vi "set_translation_style.vi"(8 "error in (no error)":errorcluster, 10 "translation style":enum16{"relative", "absolute"}(ring), 11 "StageDL090409Scaffold in":refnum<class "StageDL090409Scaffold.lvclass">) -> (0 "error out":errorcluster, 3 "StageDL090409Scaffold out":refnum<class "StageDL090409Scaffold.lvclass">)   [LabVIEW 2010, in "StageDL090409Scaffold.lvclass"]
uses:
  StageDL090409Scaffold.lvclass
  StageDL090409Scaffold.lvclass/StageDL090409Scaffold.ctl
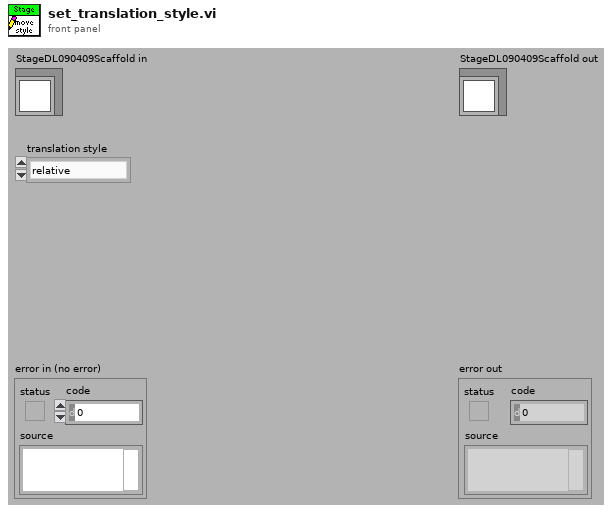
[diagram p1: front panel]
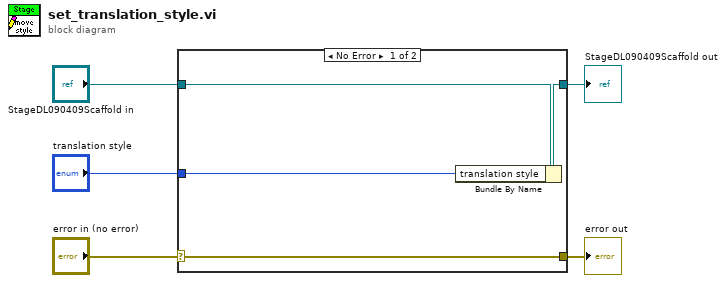
[diagram p0: block diagram]
diagram:
  n1 = case shown="No Error" "error in (no error)" {
    selector: "error in (no error)" -> [w9 w10]
    tunnel: [w9 w10] -> w4
    tunnel: [w7 w11] -> w2
    tunnel: "StageDL090409Scaffold in" -> [w8 w11]
    tunnel: "translation style" -> [w6 _]
    frame No Error {
      n2 = Bundle By Name(cluster=w8, "translation style"=w6) -> (w7:refnum<class "StageDL090409Scaffold.lvclass">)
    }
    frame Error {
    }
  }
  "error out" <- w4
  "StageDL090409Scaffold out" <- w2
